vi "Action Name.vi"(11 "SyncAction in":refnum<class "SyncAction.lvclass">) -> (2 "Action Name":string)   [LabVIEW 2020, in "GPackTools.lvlib" / "SyncAction.lvclass"]
uses:
  SyncAction.lvclass
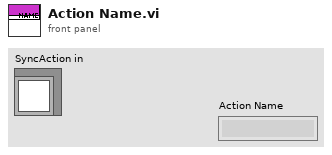
[diagram p1: front panel]
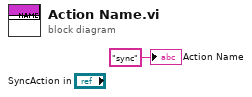
[diagram p0: block diagram]
diagram:
  "Action Name" <- "sync" ("Action Name")
